vi "UpdateCaliperToMainResultTable.vi"(7 "Type":enum16{"TagName", "Value"}(ring), 11 "ProjectName":string) -> (3 "CaliperResultNames":string[](array[string]))   [LabVIEW 2019]
uses:
  Controls/Caliper_Entry_FGV_Action.ctl
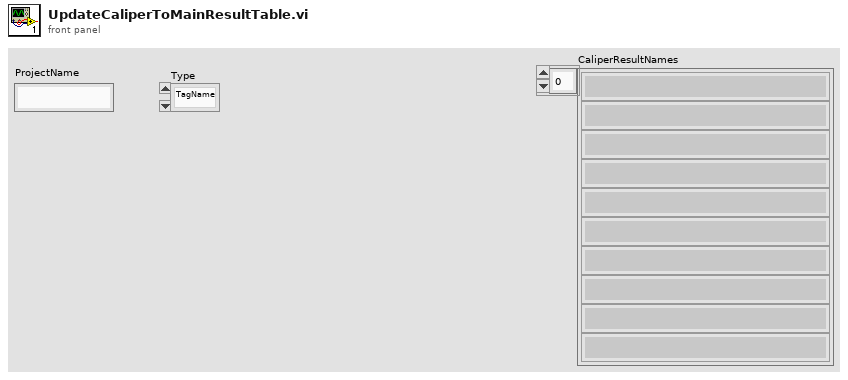
[diagram p1: front panel]
types:
  T1 = typedef "Caliper_Entry_FGV_Action.ctl" = enum16{"Init", "Close", "Add", "Delete", "ReplaceAll", "ReadAll"}
  T2 = typedef "CaliperDataEntry.ctl" = cluster{"CaliperType":T3, "Points":T4[], "Result":T6, "StepName":string}
  T3 = typedef "CaliperType.ctl" = u32
  T4 = typedef "SelectionListEntry.ctl" = cluster{"Type":T5, "Index":i32}
  T5 = typedef "SelectionListEntryPointType.ctl" = enum16{"AnalysisResult", "CaliperResult"}
  T6 = typedef "CaliperResult.ctl" = cluster{"PointInclude?":bool, "Num_Of_Pts":u8, "Position.X":dbl, "Position.Y":dbl, "Angle":dbl, "Distance":dbl, "Area":dbl, "Radius_MAX":dbl, "Radius2_min":dbl, "Dev_Residual":dbl, "P2.X":dbl, "P2.Y":dbl, "StepName":string, "Point ID":u8, "StepError?":bool, "ResultDiff?":bool}
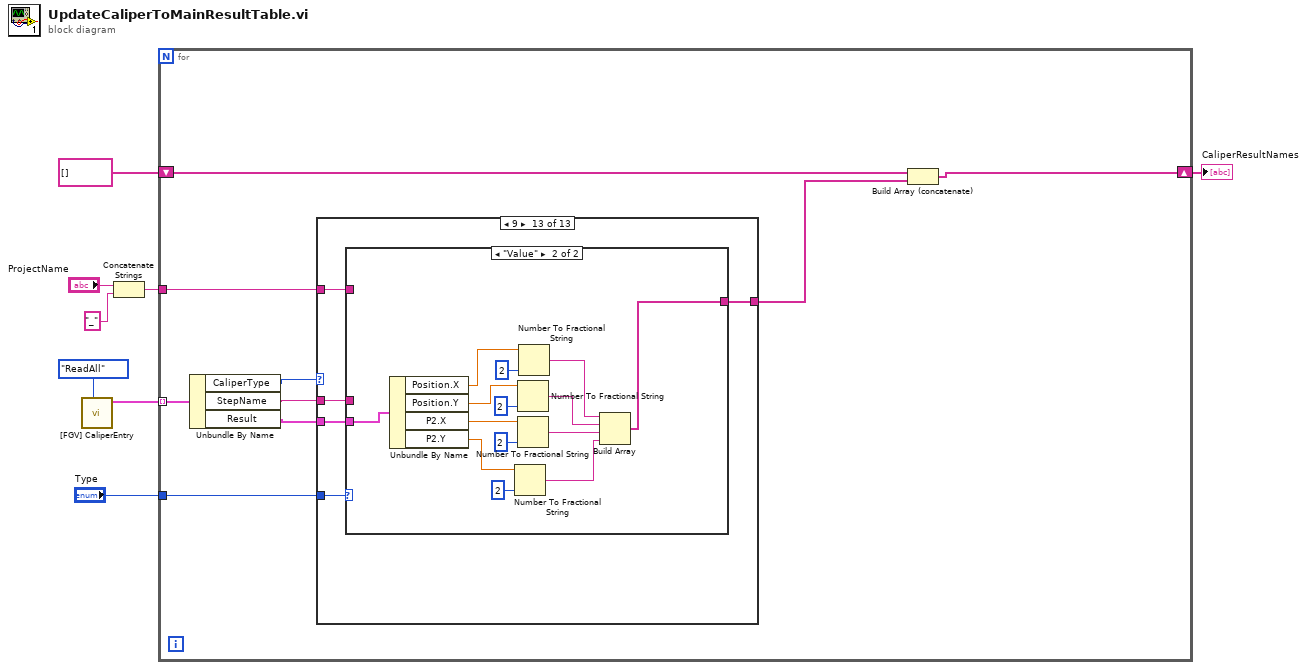
[diagram p0: block diagram]
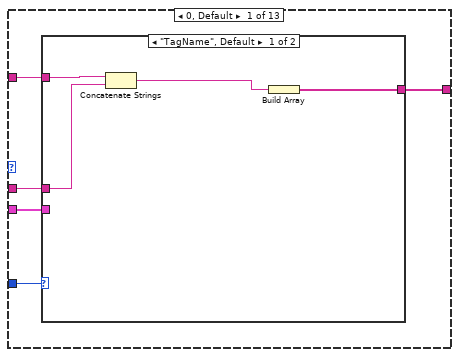
[diagram p2: hidden frame]
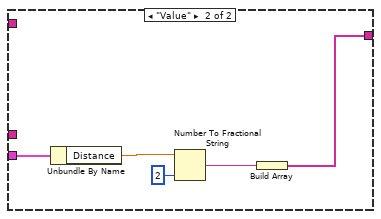
[diagram p3: hidden frame]
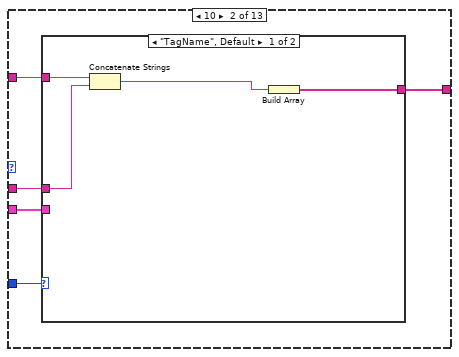
[diagram p4: hidden frame]
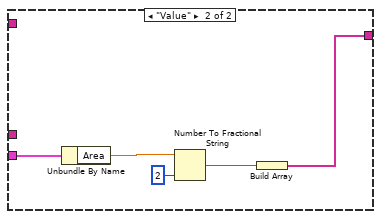
[diagram p5: hidden frame]
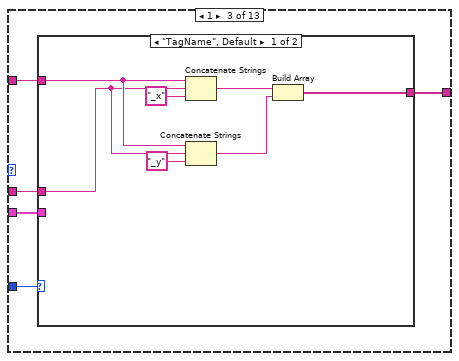
[diagram p6: hidden frame]
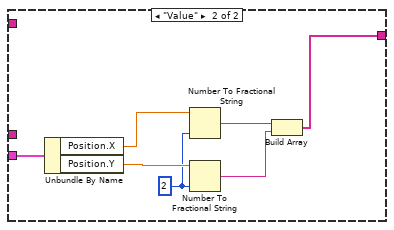
[diagram p7: hidden frame]
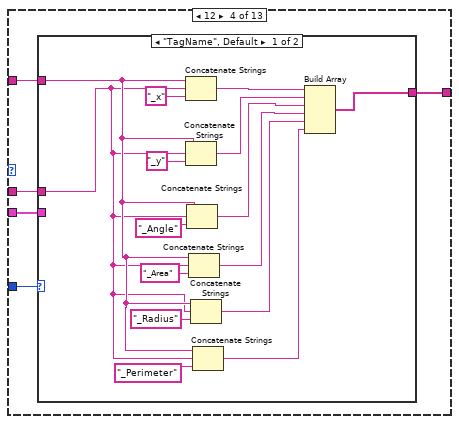
[diagram p8: hidden frame]
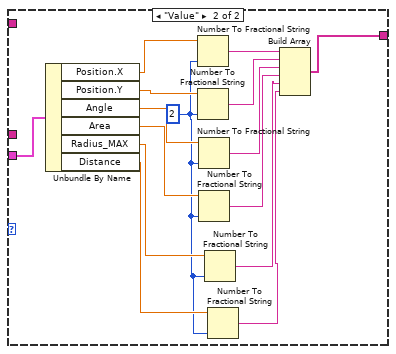
[diagram p9: hidden frame]
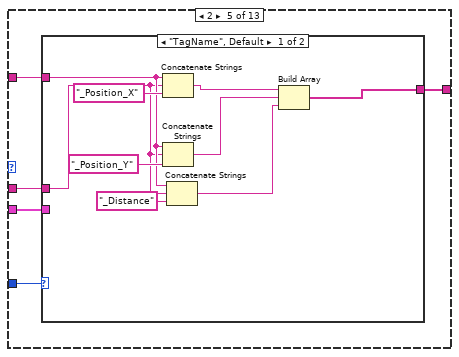
[diagram p10: hidden frame]
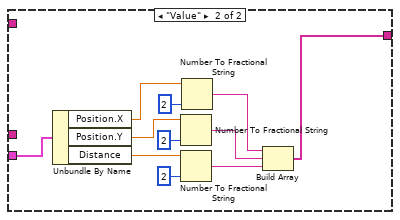
[diagram p11: hidden frame]
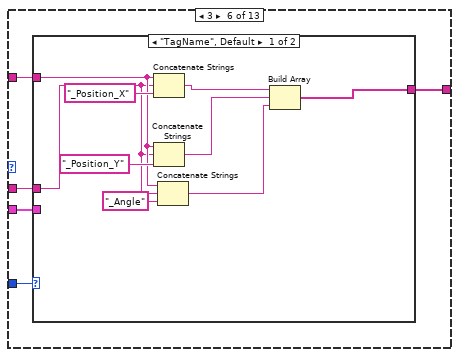
[diagram p12: hidden frame]
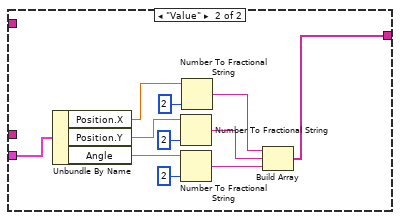
[diagram p13: hidden frame]
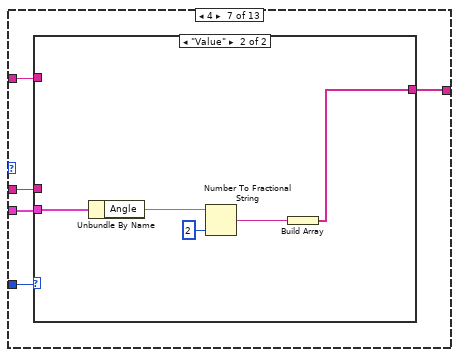
[diagram p14: hidden frame]
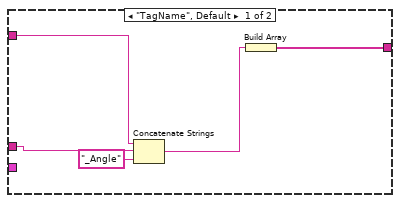
[diagram p15: hidden frame]
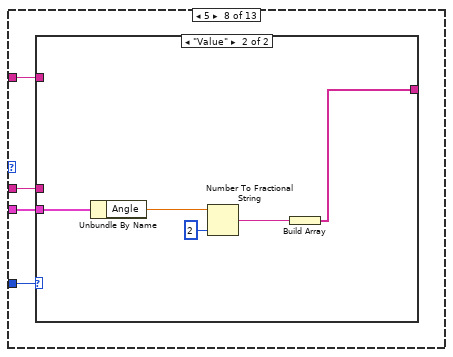
[diagram p16: hidden frame]
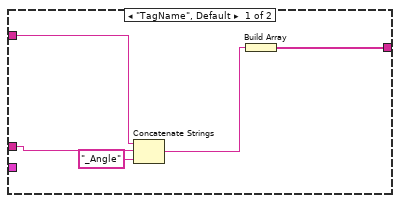
[diagram p17: hidden frame]
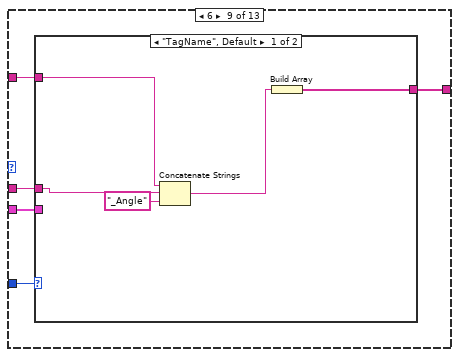
[diagram p18: hidden frame]
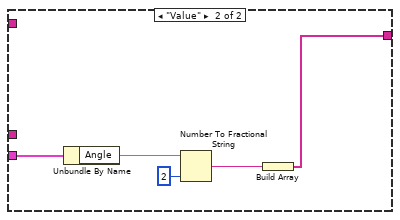
[diagram p19: hidden frame]
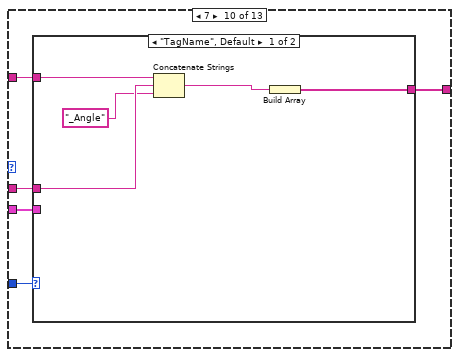
[diagram p20: hidden frame]
diagram:
  n1 = call "[FGV] CaliperEntry.vi"("Action"=Caliper_Entry_FGV_Action."ReadAll") -> ("AllCaliperEntries"=w7:T2[])  [unwired: 9 in, 1 out]
  n2 = Concatenate Strings("ProjectName", "_" ("string")) -> (w2:string)
  n3 = for {
    tunnel: w7 -> [w17] mode=indexing
    shift-right: [w11] -> w5
    shift-left: string[] [] -> [w12]
    tunnel: w2 -> [w13]
    tunnel: "Type" -> [w10]
    n4 = Unbundle By Name(w17) -> ("CaliperType"=w16:T3, "StepName"=w15:string, "Result"=w14:T6)
    n5 = case shown="9" w16 {
      tunnel: w15 -> [w21 w35 w49 w68 w101 w128 w151 w167 w182 w197 w211 w241 w275]
      tunnel: w14 -> [w18 w32 w46 w65 w102 w125 w152 w166 w181 w194 w210 w240 w274]
      tunnel: w13 -> [w22 w36 w50 w69 w103 w129 w153 w168 w183 w198 w212 w242 w276]
      tunnel: [w20 w34 w48 w67 w104 w127 w154 _ w180 w196 _ w238 w277] -> w9
      tunnel: w10 -> [w19 w33 w47 w66 w100 w126 w150 w165 w179 w195 w209 w239 w273]
      frame 0, Default {
        n6 = case shown="\"TagName\", Default" w19 {
          tunnel: w22 -> [w26 _]
          tunnel: w21 -> [w25 _]
          tunnel: [w23 w27] -> w20
          tunnel: w18 -> [_ w31]
          frame "TagName", Default {
            n7 = Concatenate Strings(w26, w25) -> (w24:string)
            n8 = Build Array(w24) -> (w23:string[])
          }
          frame "Value" {
            n9 = Unbundle By Name(w31) -> ("Distance"=w30:dbl)
            n10 = Number To Fractional String(number=w30, precision (6)=i16 2) -> (F-format string=w28:string)  [unwired: 2 in]
            n11 = Build Array(w28) -> (w27:string[])
          }
        }
      }
      frame 10 {
        n12 = case shown="\"TagName\", Default" w33 {
          tunnel: w36 -> [w40 _]
          tunnel: w35 -> [w39 _]
          tunnel: [w37 w41] -> w34
          tunnel: w32 -> [_ w45]
          frame "TagName", Default {
            n13 = Concatenate Strings(w40, w39) -> (w38:string)
            n14 = Build Array(w38) -> (w37:string[])
          }
          frame "Value" {
            n15 = Unbundle By Name(w45) -> ("Area"=w44:dbl)
            n16 = Number To Fractional String(number=w44, precision (6)=i16 2) -> (F-format string=w42:string)  [unwired: 2 in]
            n17 = Build Array(w42) -> (w41:string[])
          }
        }
      }
      frame 1 {
        n18 = case shown="\"TagName\", Default" w47 {
          tunnel: w50 -> [w57 _]
          tunnel: w49 -> [w56 _]
          tunnel: [w51 w58] -> w48
          tunnel: w46 -> [_ w64]
          frame "TagName", Default {
            n19 = Concatenate Strings(w57, w56, "_x" ("string")) -> (w53:string)
            n20 = Concatenate Strings(w57, w56, "_y" ("string")) -> (w52:string)
            n21 = Build Array(w53, w52) -> (w51:string[])
          }
          frame "Value" {
            w59 = i16 2 ("precision (6)")
            n22 = Unbundle By Name(w64) -> ("Position.X"=w61:dbl, "Position.Y"=w60:dbl)
            n23 = Number To Fractional String(number=w61, precision (6)=w59) -> (F-format string=w63:string)  [unwired: 2 in]
            n24 = Number To Fractional String(number=w60, precision (6)=w59) -> (F-format string=w62:string)  [unwired: 2 in]
            n25 = Build Array(w63, w62) -> (w58:string[])
          }
        }
      }
      frame 12 {
        n26 = case shown="\"TagName\", Default" w66 {
          tunnel: w69 -> [w75 _]
          tunnel: w68 -> [w74 _]
          tunnel: [w80 w94] -> w67
          tunnel: w65 -> [_ w99]
          frame "TagName", Default {
            n27 = Concatenate Strings(w75, w74, "_x" ("string")) -> (w82:string)
            n28 = Concatenate Strings(w75, w74, "_y" ("string")) -> (w81:string)
            n29 = Concatenate Strings(w75, w74, "_Angle" ("string")) -> (w73:string)
            n30 = Concatenate Strings(w75, w74, "_Area" ("string")) -> (w72:string)
            n31 = Concatenate Strings(w75, w74, "_Radius" ("string")) -> (w71:string)
            n32 = Concatenate Strings(w75, w74, "_Perimeter" ("string")) -> (w70:string)
            n33 = Build Array(w82, w81, w73, w72, w71, w70) -> (w80:string[])
          }
          frame "Value" {
            w89 = i16 2 ("precision (6)")
            n34 = Unbundle By Name(w99) -> ("Position.X"=w96:dbl, "Position.Y"=w95:dbl, "Angle"=w93:dbl, "Area"=w92:dbl, "Radius_MAX"=w91:dbl, "Distance"=w90:dbl)
            n35 = Number To Fractional String(number=w96, precision (6)=w89) -> (F-format string=w98:string)  [unwired: 2 in]
            n36 = Number To Fractional String(number=w95, precision (6)=w89) -> (F-format string=w97:string)  [unwired: 2 in]
            n37 = Number To Fractional String(number=w93, precision (6)=w89) -> (F-format string=w88:string)  [unwired: 2 in]
            n38 = Number To Fractional String(number=w92, precision (6)=w89) -> (F-format string=w87:string)  [unwired: 2 in]
            n39 = Number To Fractional String(number=w91, precision (6)=w89) -> (F-format string=w86:string)  [unwired: 2 in]
            n40 = Number To Fractional String(number=w90, precision (6)=w89) -> (F-format string=w85:string)  [unwired: 2 in]
            n41 = Build Array(w98, w97, w88, w87, w86, w85) -> (w94:string[])
          }
        }
      }
      frame 2 {
        n42 = case shown="\"TagName\", Default" w100 {
          tunnel: w103 -> [w108 _]
          tunnel: w101 -> [w107 _]
          tunnel: [w113 w120] -> w104
          tunnel: w102 -> [_ w121]
          frame "TagName", Default {
            n43 = Concatenate Strings(w108, w107, "_Position_X" ("string")) -> (w110:string)
            n44 = Concatenate Strings(w108, w107, "_Position_Y" ("string")) -> (w109:string)
            n45 = Concatenate Strings(w108, w107, "_Distance" ("string")) -> (w105:string)
            n46 = Build Array(w110, w109, w105) -> (w113:string[])
          }
          frame "Value" {
            n47 = Unbundle By Name(w121) -> ("Position.X"=w117:dbl, "Position.Y"=w116:dbl, "Distance"=w124:dbl)
            n48 = Number To Fractional String(number=w116, precision (6)=i16 2) -> (F-format string=w114:string)  [unwired: 2 in]
            n49 = Number To Fractional String(number=w124, precision (6)=i16 2) -> (F-format string=w122:string)  [unwired: 2 in]
            n50 = Number To Fractional String(number=w117, precision (6)=i16 2) -> (F-format string=w115:string)  [unwired: 2 in]
            n51 = Build Array(w115, w114, w122) -> (w120:string[])
          }
        }
      }
      frame 3 {
        n52 = case shown="\"TagName\", Default" w126 {
          tunnel: w129 -> [w133 _]
          tunnel: w128 -> [w132 _]
          tunnel: [w138 w145] -> w127
          tunnel: w125 -> [_ w146]
          frame "TagName", Default {
            n53 = Concatenate Strings(w133, w132, "_Position_X" ("string")) -> (w135:string)
            n54 = Concatenate Strings(w133, w132, "_Position_Y" ("string")) -> (w134:string)
            n55 = Concatenate Strings(w133, w132, "_Angle" ("string")) -> (w130:string)
            n56 = Build Array(w135, w134, w130) -> (w138:string[])
          }
          frame "Value" {
            n57 = Unbundle By Name(w146) -> ("Position.X"=w142:dbl, "Position.Y"=w141:dbl, "Angle"=w149:dbl)
            n58 = Number To Fractional String(number=w141, precision (6)=i16 2) -> (F-format string=w139:string)  [unwired: 2 in]
            n59 = Number To Fractional String(number=w149, precision (6)=i16 2) -> (F-format string=w147:string)  [unwired: 2 in]
            n60 = Number To Fractional String(number=w142, precision (6)=i16 2) -> (F-format string=w140:string)  [unwired: 2 in]
            n61 = Build Array(w140, w139, w147) -> (w145:string[])
          }
        }
      }
      frame 4 {
        n62 = case shown="\"Value\"" w150 {
          tunnel: w153 -> [w156 _]
          tunnel: w151 -> [w155 _]
          tunnel: [w159 w160] -> w154
          tunnel: w152 -> [_ w161]
          frame "TagName", Default {
            n63 = Concatenate Strings(w156, w155, "_Angle" ("string")) -> (w157:string)
            n64 = Build Array(w157) -> (w159:string[])
          }
          frame "Value" {
            n65 = Unbundle By Name(w161) -> ("Angle"=w164:dbl)
            n66 = Number To Fractional String(number=w164, precision (6)=i16 2) -> (F-format string=w162:string)  [unwired: 2 in]
            n67 = Build Array(w162) -> (w160:string[])
          }
        }
      }
      frame 5 {
        n68 = case shown="\"Value\"" w165 {
          tunnel: w168 -> [w170 _]
          tunnel: w167 -> [w169 _]
          tunnel: [w173 w174] -> _
          tunnel: w166 -> [_ w175]
          frame "TagName", Default {
            n69 = Concatenate Strings(w170, w169, "_Angle" ("string")) -> (w171:string)
            n70 = Build Array(w171) -> (w173:string[])
          }
          frame "Value" {
            n71 = Unbundle By Name(w175) -> ("Angle"=w178:dbl)
            n72 = Number To Fractional String(number=w178, precision (6)=i16 2) -> (F-format string=w176:string)  [unwired: 2 in]
            n73 = Build Array(w176) -> (w174:string[])
          }
        }
      }
      frame 6 {
        n74 = case shown="\"TagName\", Default" w179 {
          tunnel: w183 -> [w185 _]
          tunnel: w182 -> [w184 _]
          tunnel: [w188 w189] -> w180
          tunnel: w181 -> [_ w190]
          frame "TagName", Default {
            n75 = Concatenate Strings(w185, w184, "_Angle" ("string")) -> (w186:string)
            n76 = Build Array(w186) -> (w188:string[])
          }
          frame "Value" {
            n77 = Unbundle By Name(w190) -> ("Angle"=w193:dbl)
            n78 = Number To Fractional String(number=w193, precision (6)=i16 2) -> (F-format string=w191:string)  [unwired: 2 in]
            n79 = Build Array(w191) -> (w189:string[])
          }
        }
      }
      frame 7 {
        n80 = case shown="\"TagName\", Default" w195 {
          tunnel: w198 -> [w203 _]
          tunnel: w197 -> [w202 _]
          tunnel: [w200 w204] -> w196
          tunnel: w194 -> [_ w205]
          frame "TagName", Default {
            n81 = Concatenate Strings(w203, w202, "_Angle" ("string")) -> (w201:string)
            n82 = Build Array(w201) -> (w200:string[])
          }
          frame "Value" {
            n83 = Unbundle By Name(w205) -> ("Angle"=w208:dbl)
            n84 = Number To Fractional String(number=w208, precision (6)=i16 2) -> (F-format string=w206:string)  [unwired: 2 in]
            n85 = Build Array(w206) -> (w204:string[])
          }
        }
      }
      frame 8 {
        n86 = case shown="\"TagName\", Default" w209 {
          tunnel: w212 -> [w214 _]
          tunnel: w211 -> [w213 _]
          tunnel: [w223 w234] -> _
          tunnel: w210 -> [_ w235]
          frame "TagName", Default {
            n87 = Concatenate Strings(w214, w213, "_Position1_X" ("string")) -> (w220:string)
            n88 = Concatenate Strings(w214, w213, "_Position1_Y" ("string")) -> (w219:string)
            n89 = Concatenate Strings(w214, w213, "_Position2_X" ("string")) -> (w217:string)
            n90 = Concatenate Strings(w214, w213, "_Position2_Y" ("string")) -> (w215:string)
            n91 = Build Array(w220, w219, w217, w215) -> (w223:string[])
          }
          frame "Value" {
            n92 = Unbundle By Name(w235) -> ("Position.X"=w231:dbl, "Position.Y"=w230:dbl, "P2.X"=w237:dbl, "P2.Y"=w225:dbl)
            n93 = Number To Fractional String(number=w225, precision (6)=i16 2) -> (F-format string=w224:string)  [unwired: 2 in]
            n94 = Number To Fractional String(number=w230, precision (6)=i16 2) -> (F-format string=w228:string)  [unwired: 2 in]
            n95 = Number To Fractional String(number=w237, precision (6)=i16 2) -> (F-format string=w236:string)  [unwired: 2 in]
            n96 = Number To Fractional String(number=w231, precision (6)=i16 2) -> (F-format string=w229:string)  [unwired: 2 in]
            n97 = Build Array(w229, w228, w236, w224) -> (w234:string[])
          }
        }
      }
      frame 11 {
        n98 = case shown="\"Value\"" w239 {
          tunnel: w242 -> [w245 _]
          tunnel: w241 -> [w244 _]
          tunnel: [w255 w269] -> w238
          tunnel: w240 -> [_ w270]
          frame "TagName", Default {
            n99 = Concatenate Strings(w245, w244, "_Position1_X" ("string")) -> (w252:string)
            n100 = Concatenate Strings(w245, w244, "_Position1_Y" ("string")) -> (w251:string)
            n101 = Concatenate Strings(w245, w244, "_Position2_X" ("string")) -> (w249:string)
            n102 = Concatenate Strings(w245, w244, "_Position2_Y" ("string")) -> (w247:string)
            n103 = Concatenate Strings(w245, w244, "_Residual" ("string")) -> (w243:string)
            n104 = Build Array(w252, w251, w249, w247, w243) -> (w255:string[])
          }
          frame "Value" {
            n105 = Unbundle By Name(w270) -> ("Position.X"=w266:dbl, "Position.Y"=w265:dbl, "P2.X"=w272:dbl, "P2.Y"=w260:dbl, "Radius_MAX"=w258:dbl)
            n106 = Number To Fractional String(number=w258, precision (6)=i16 2) -> (F-format string=w256:string)  [unwired: 2 in]
            n107 = Number To Fractional String(number=w260, precision (6)=i16 2) -> (F-format string=w259:string)  [unwired: 2 in]
            n108 = Number To Fractional String(number=w265, precision (6)=i16 2) -> (F-format string=w263:string)  [unwired: 2 in]
            n109 = Number To Fractional String(number=w272, precision (6)=i16 2) -> (F-format string=w271:string)  [unwired: 2 in]
            n110 = Number To Fractional String(number=w266, precision (6)=i16 2) -> (F-format string=w264:string)  [unwired: 2 in]
            n111 = Build Array(w264, w263, w271, w259, w256) -> (w269:string[])
          }
        }
      }
      frame 9 {
        n112 = case shown="\"Value\"" w273 {
          tunnel: w276 -> [w279 _]
          tunnel: w275 -> [w278 _]
          tunnel: [w288 w299] -> w277
          tunnel: w274 -> [_ w300]
          frame "TagName", Default {
            n113 = Concatenate Strings(w279, w278, "_Position1_X" ("string")) -> (w285:string)
            n114 = Concatenate Strings(w279, w278, "_Position1_Y" ("string")) -> (w284:string)
            n115 = Concatenate Strings(w279, w278, "_Position2_X" ("string")) -> (w282:string)
            n116 = Concatenate Strings(w279, w278, "_Position2_Y" ("string")) -> (w280:string)
            n117 = Build Array(w285, w284, w282, w280) -> (w288:string[])
          }
          frame "Value" {
            n118 = Unbundle By Name(w300) -> ("Position.X"=w296:dbl, "Position.Y"=w295:dbl, "P2.X"=w302:dbl, "P2.Y"=w290:dbl)
            n119 = Number To Fractional String(number=w290, precision (6)=i16 2) -> (F-format string=w289:string)  [unwired: 2 in]
            n120 = Number To Fractional String(number=w295, precision (6)=i16 2) -> (F-format string=w293:string)  [unwired: 2 in]
            n121 = Number To Fractional String(number=w302, precision (6)=i16 2) -> (F-format string=w301:string)  [unwired: 2 in]
            n122 = Number To Fractional String(number=w296, precision (6)=i16 2) -> (F-format string=w294:string)  [unwired: 2 in]
            n123 = Build Array(w294, w293, w301, w289) -> (w299:string[])
          }
        }
      }
    }
    n124 = Build Array (concatenate)(w12, w9) -> (w11:string[])
  }
  "CaliperResultNames" <- w5
